vi "linkam.exit.vi"(8 "error in (no error)":errorcluster, 11 "VISA resource name in":refnum<visa-resource-name>) -> (0 "error out":errorcluster, 3 "VISA resource name out":refnum<visa-resource-name>)   [LabVIEW 8.6]
panel:
  in  "Serial Settings:Number of Bytes at Serial Port":u32
  in  "write":string
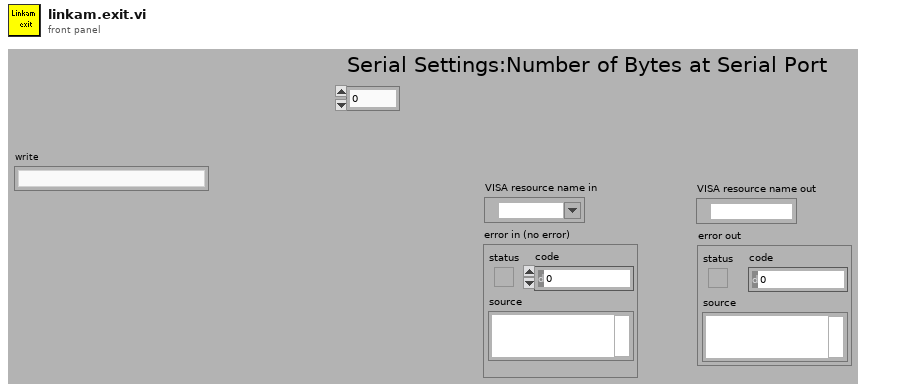
[diagram p1: front panel]
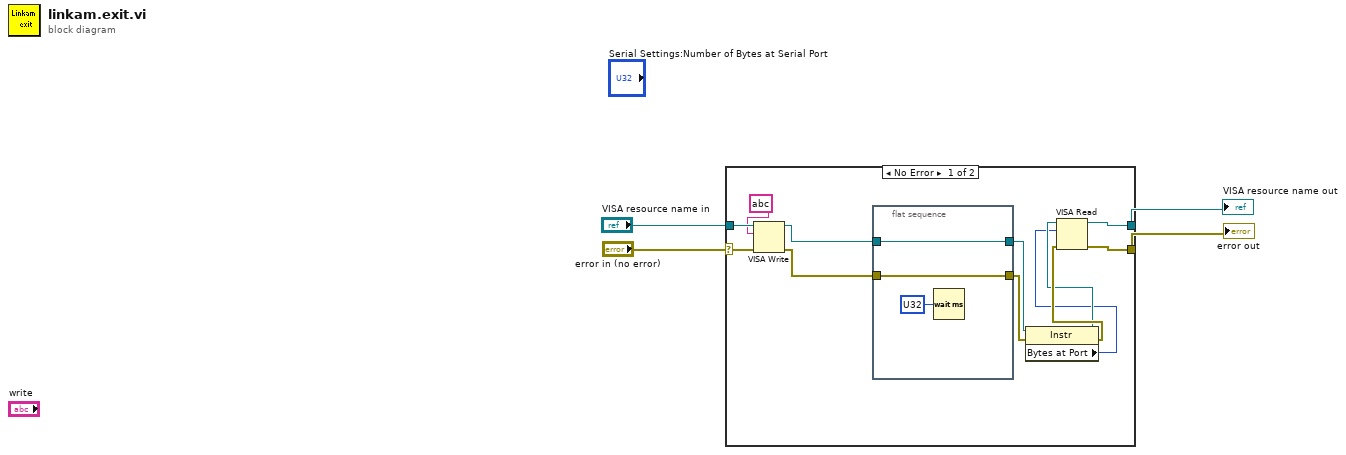
[diagram p0: block diagram]
diagram:
  n1 = case shown="No Error" "error in (no error)" {
    selector: "error in (no error)" -> [w15 w21]
    tunnel: [w13 w21] -> w3
    tunnel: [w14 w20] -> w4
    tunnel: "VISA resource name in" -> [w16 w20]
    frame #0 {
      n2 = VISA Write(VISA resource name=w16, write buffer=string ?, error in (no error)=w15) -> (VISA resource name out=w11:refnum<visa-resource-name>, error out=w10:errorcluster)  [unwired: 1 out]
      n3 = flat-sequence {
        tunnel: w11 -> [w18]
        tunnel: [w18] -> w7
        tunnel: w10 -> [w17]
        tunnel: [w17] -> w6
        frame #0 {
          n4 = Wait (ms)(milliseconds to wait=u32 ?) -> ()  [unwired: 1 out]
        }
      }
      n5 = property class="Instr"(reference=w7, error in=w6) -> (reference out=w8:refnum<visa-resource-name>, error out=w9:errorcluster, "Bytes at Port"=w5:u32)
      n6 = VISA Read(VISA resource name=w8, byte count=w5, error in (no error)=w9) -> (VISA resource name out=w14:refnum<visa-resource-name>, error out=w13:errorcluster)  [unwired: 2 out]
    }
    frame #1 {
    }
  }
  "VISA resource name out" <- w4
  "error out" <- w3
